vi "Read Destination path.vi"(11 "ProjectItem in":refnum<class "ProjectItem.lvclass">) -> (2 "Destination path":path, 3 "ProjectItem out":refnum<class "ProjectItem.lvclass">)   [LabVIEW 2019, in "SolutionBuilder.lvlib" / "ProjectItem.lvclass"]
uses:
  ProjectItem.lvclass
  ProjectItem.lvclass/ProjectItem.ctl
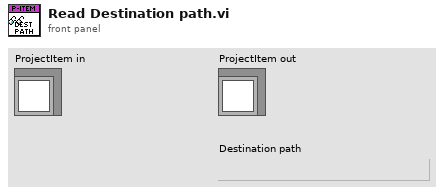
[diagram p1: front panel]
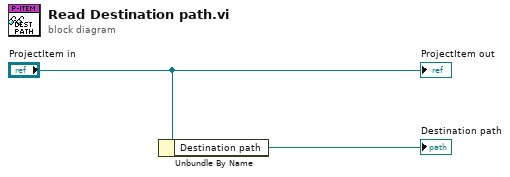
[diagram p0: block diagram]
diagram:
  n1 = Unbundle By Name("ProjectItem in") -> ("Destination path"=→"Destination path":path)
  "ProjectItem out" <- "ProjectItem in"
